vi "Change Font.vi"(8 "error in (no error)":errorcluster, 11 "Filled Text Fields Actor in":refnum<class "Filled Text Fields Actor.lvclass">) -> (0 "error out":errorcluster, 3 "Filled Text Fields Actor out":refnum<class "Filled Text Fields Actor.lvclass">)   [LabVIEW 2017, in "Filled Text Fields Actor.lvlib" / "Filled Text Fields Actor.lvclass"]
uses:
  Filled Text Fields Actor.lvclass
  Filled Text Fields Actor.lvclass/Filled Text Fields Actor.ctl
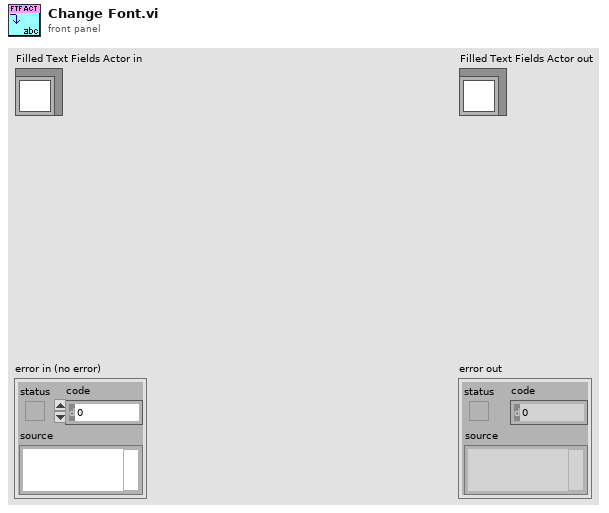
[diagram p1: front panel]
types:
  T1 = typedef "Theme.lvlib/Theme.Font.lvclass/Font.ctl" = cluster{"Size":u32, "Shrink Size":u32, "Name":string, "Password Display":bool}
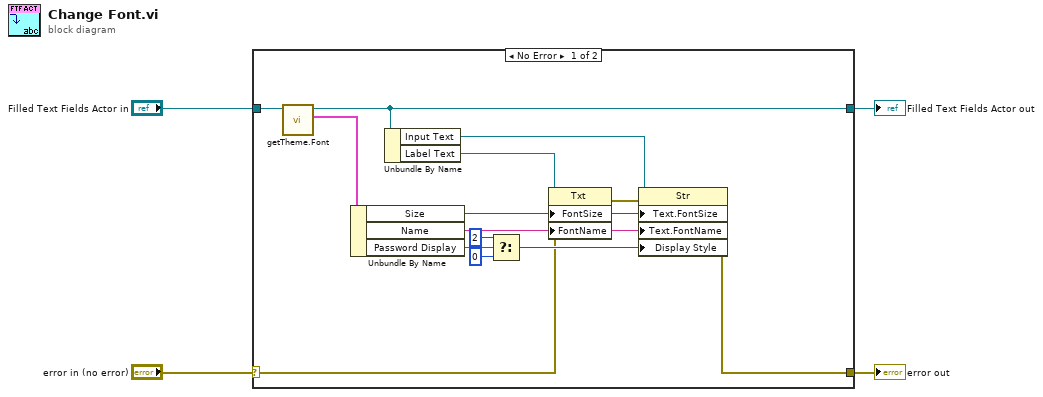
[diagram p0: block diagram]
diagram:
  n1 = case shown="No Error" "error in (no error)" {
    selector: "error in (no error)" -> [w6 w20]
    tunnel: [w5 w20] -> w3
    tunnel: [w17 w19] -> w1
    tunnel: "Filled Text Fields Actor in" -> [w18 w19]
    frame No Error {
      n2 = call "getTheme.Font.vi"("Filled Text Fields Actor in"=w18) -> ("Font"=w15:T1, "Filled Text Fields Actor out"=w17:refnum<class "Filled Text Fields Actor.lvclass">)  [unwired: 9 in]
      n3 = Unbundle By Name(w15) -> ("Size"=w9:u32, "Name"=w8:string, "Password Display"=w12:bool)
      n4 = Unbundle By Name(w17) -> ("Input Text"=w16:refnum<vi>, "Label Text"=w10:refnum<vi>)
      n5 = Select(t=u32 2 ("Display Style"), s=w12, f=u32 0) -> (s? t:f=w11:u32)
      n6 = property class="Txt"(reference=w10, error in=w6, "FontSize"=w9, "FontName"=w8) -> (error out=w7:errorcluster)  [unwired: 1 out]
      n7 = property class="Str"(reference=w16, error in=w7, "Text.FontSize"=w9, "Text.FontName"=w8, "Display Style"=w11) -> (error out=w5:errorcluster)  [unwired: 1 out]
    }
    frame Error {
    }
  }
  "error out" <- w3
  "Filled Text Fields Actor out" <- w1
